vi "DataTrcFileRichInfo.vi"(9 "Language":u32, 11 "file path (dialog if empty)":path caption="文件路径 （空时为对话框）") -> (0 "路径输出":path, 1 "FileInfo":string, 2 "文件类型":string)   [LabVIEW 2015]
uses:
  <vilib>/Utility/file.llb/Read Delimited Spreadsheet (string).vi
  <vilib>/regexp/Match Regular Expression.xnode
panel:
  out "总帧数":i32
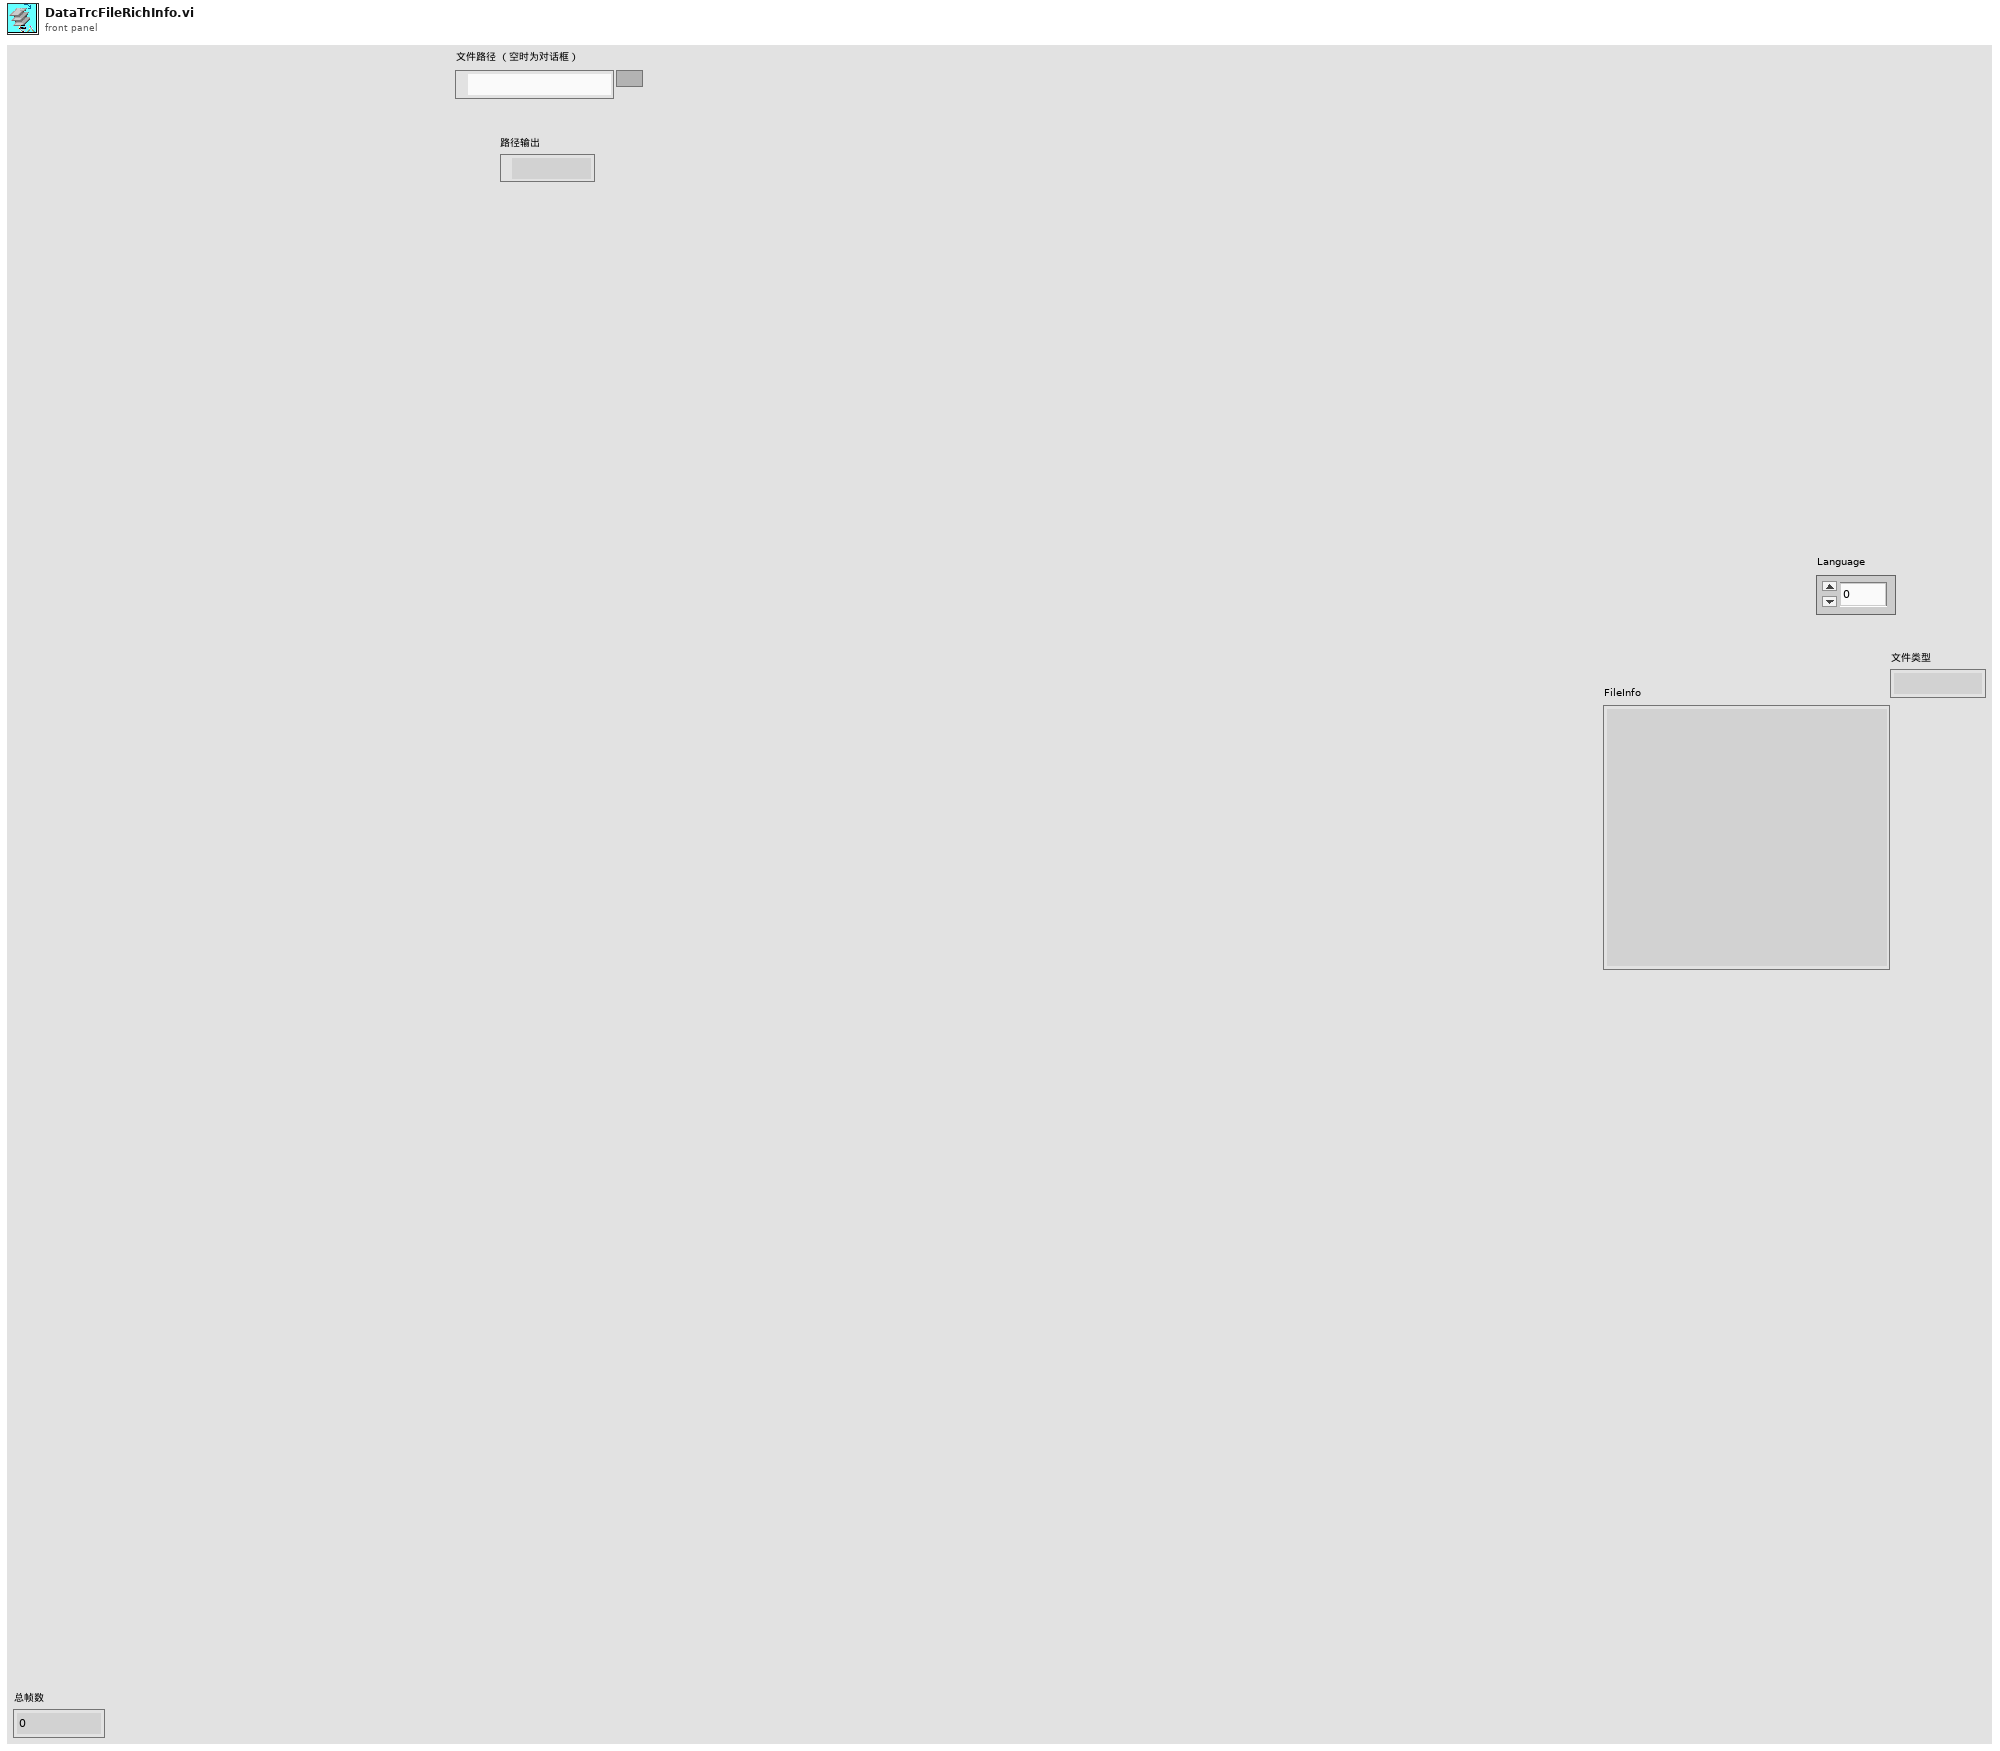
[diagram p1: front panel]
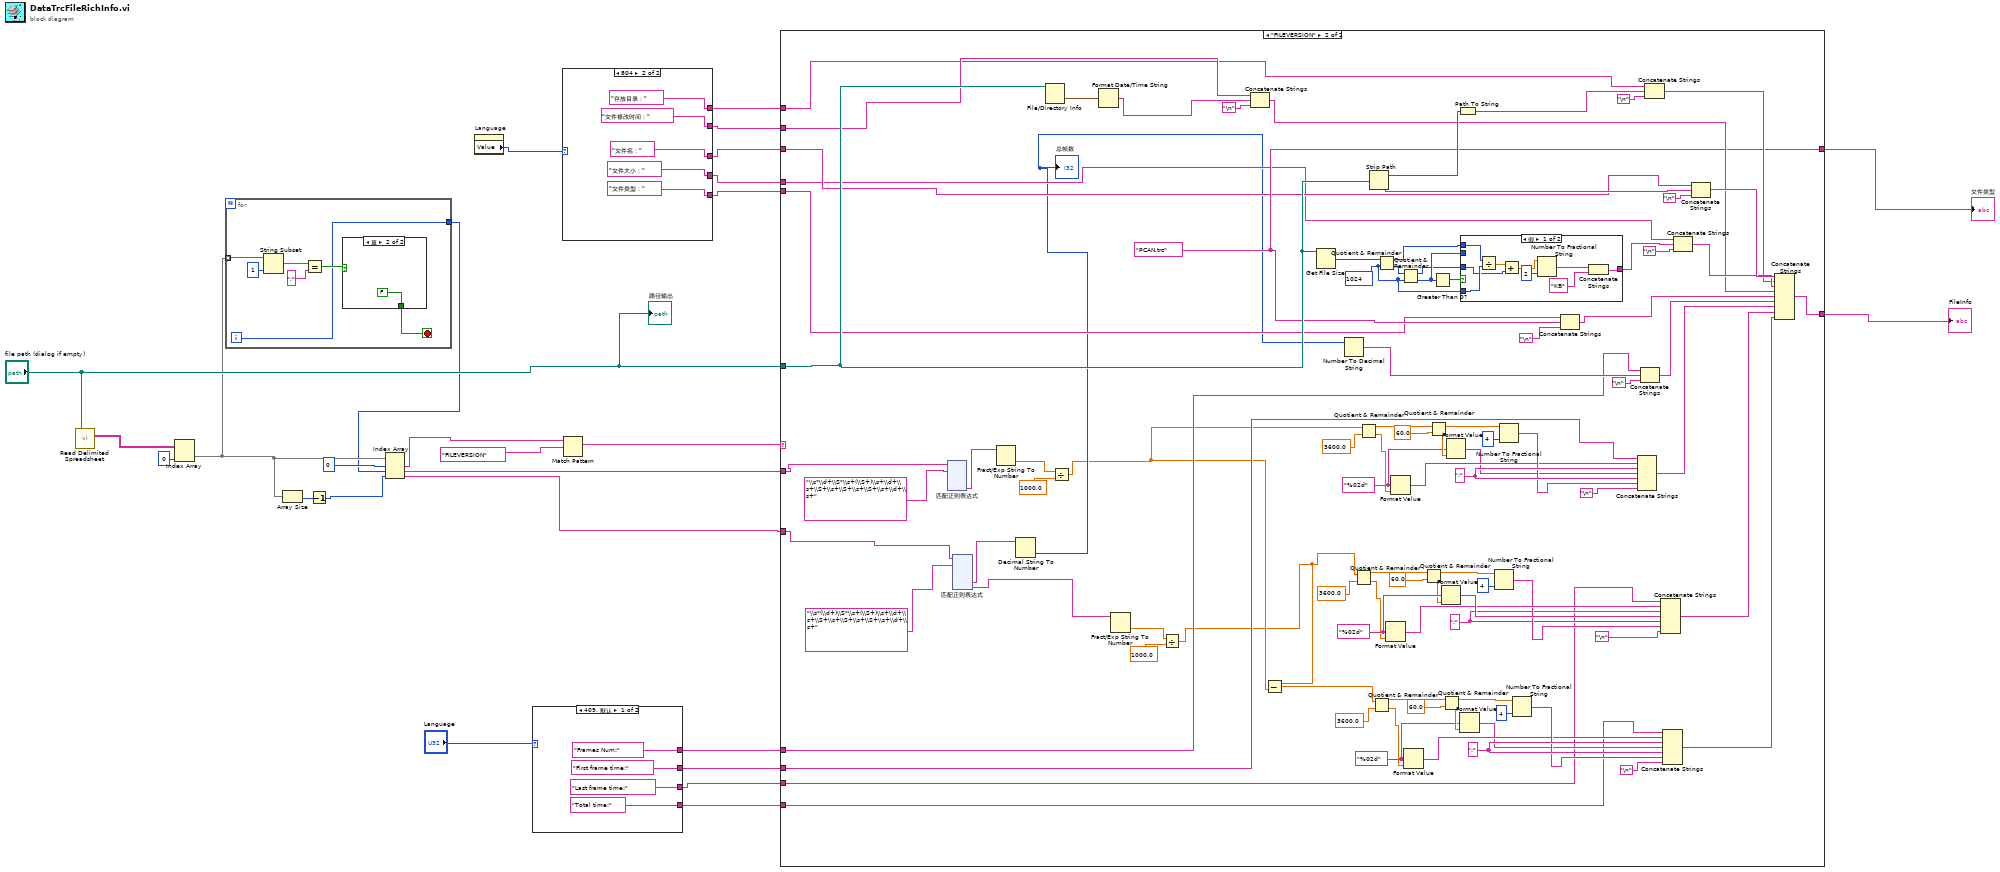
[diagram p0: block diagram]
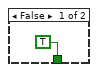
[diagram p2: hidden frame]
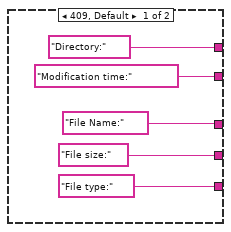
[diagram p3: hidden frame]
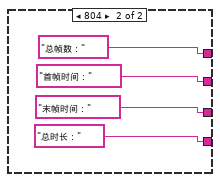
[diagram p4: hidden frame]
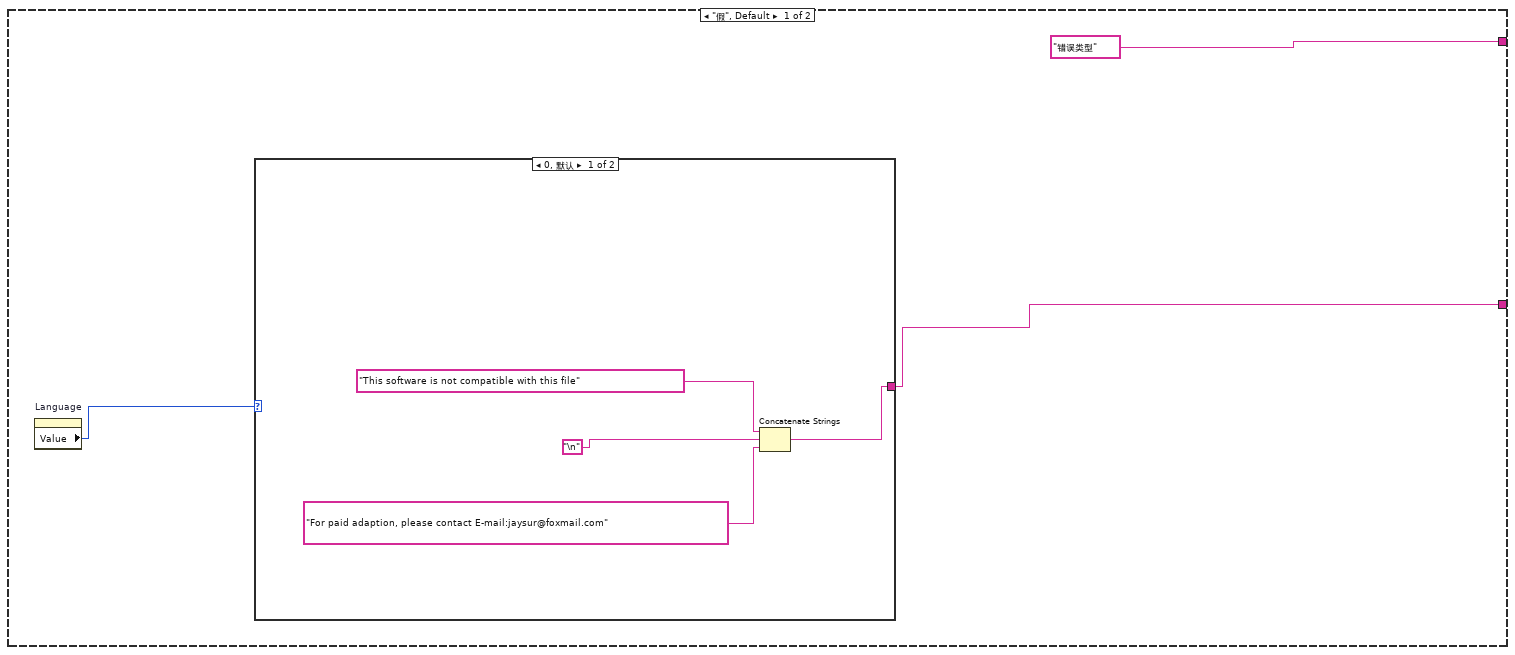
[diagram p5: hidden frame]
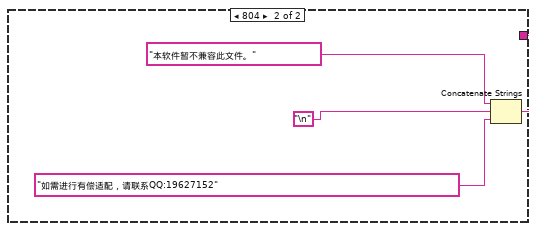
[diagram p6: hidden frame]
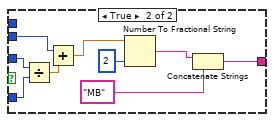
[diagram p7: hidden frame]
diagram:
  n1 = call-poly <vilib>:"Read Delimited Spreadsheet.vi"("file path (dialog if empty)"="file path (dialog if empty)") -> ("all rows"=w12:string[][])  [unwired: 9 in, 5 out]
  n2 = Index Array(array=w12, index (col)=0 ("禁用的索引 (列)")) -> (element=w3:string[])  [unwired: 1 in]
  n3 = for {
    tunnel: w3 -> [w33] mode=indexing
    tunnel: [w27] -> w2
    i -> [w27]
    stop <- w28 stop-if-true
    n4 = String Subset(string=w33, length (rest)=1 ("长度（剩余）")) -> (substring=w31:string)  [unwired: 1 in]
    n5 = Equal?(x=w31, y=";") -> (x = y?=w29:bool)
    n6 = case shown="真" w29 {
      tunnel: [TRUE FALSE] -> w28
      frame False {
      }
      frame True {
      }
    }
  }
  n7 = Array Size(array=w3) -> (size(s)=w11:i32)
  n8 = Decrement(x=w11) -> (x-1=w9:i32)
  n9 = Index Array(array=w3, index #1=0, index #2=w2, index #3=w9) -> (element #1=w7:string, element #2=w5:string, element #3=w4:string)
  n10 = property on="Language" class="DigNum (严格)"() -> ("Value"=w23:u32)  [unwired: 2 in, 2 out]
  n11 = case shown="409, 默认" "Language" {
    tunnel: ["Total time:" "总时长："] -> w17
    tunnel: ["Last frame time:" "末帧时间："] -> w16
    tunnel: ["First frame time:" "首帧时间："] -> w15
    tunnel: ["Frames Num:" "总帧数："] -> w14
    frame 409, Default {
    }
    frame 804 {
    }
  }
  n12 = case shown="804" w23 {
    tunnel: ["Modification time:" "文件修改时间："] -> w22
    tunnel: ["Directory:" "存放目录："] -> w19
    tunnel: ["File Name:" "文件名："] -> w20
    tunnel: ["File size:" "文件大小："] -> w18
    tunnel: ["File type:" "文件类型："] -> w21
    frame 409, Default {
    }
    frame 804 {
    }
  }
  n13 = Match Pattern(string=w7, regular expression="FILEVERSION" ("正则表达式")) -> (match substring=w6:string)  [unwired: 1 in, 3 out]
  n14 = case shown="\"FILEVERSION\"" w6 {
    tunnel: ["错误类型" w87] -> w26
    tunnel: [w55 w147] -> w25
    tunnel: "file path (dialog if empty)" -> [_ w90]
    tunnel: w22 -> [_ w88]
    tunnel: w21 -> [_ w86]
    tunnel: w20 -> [_ w85]
    tunnel: w19 -> [_ w84]
    tunnel: w18 -> [_ w83]
    tunnel: w17 -> [_ w82]
    tunnel: w16 -> [_ w81]
    tunnel: w15 -> [_ w80]
    tunnel: w14 -> [_ w79]
    tunnel: w5 -> [_ w77]
    tunnel: w4 -> [_ w78]
    frame "假", Default {
      n15 = property on="Language" class="DigNum (严格)"() -> ("Value"=w54:u32)  [unwired: 2 in, 2 out]
      n16 = case shown="0, 默认" w54 {
        tunnel: [w57 w61] -> w55
        frame 0, Default {
          n17 = Concatenate Strings("This software is not compatible with this file", "\n", "For paid adaption, please contact E-mail:jaysur@foxmail.com") -> (w57:string)
        }
        frame 804 {
          n18 = Concatenate Strings("本软件暂不兼容此文件。", "\n", "如需进行有偿适配，请联系QQ:19627152") -> (w61:string)
        }
      }
    }
    frame "FILEVERSION" {
      w87 = "PCAN.trc"
      w102 = i64 1024 ("y")
      w121 = "%02d" ("格式字符串")
      w127 = ":"
      w145 = "%02d" ("格式字符串")
      w139 = ":"
      w148 = "%02d" ("格式字符串")
      w154 = ":"
      n19 = xnode "匹配正则表达式"("输入字符串"=w77, "正则表达式"="\\s*\\d+\\S*\\s+(\\S+)\\s+\\d+\\s+\\S+\\s+\\S+\\s+\\S+\\s+\\d+\\s+" ("格式字符串")) -> ("子匹配 1"=w76:string)  [unwired: 4 in, 5 out]
      n20 = xnode "匹配正则表达式"("输入字符串"=w78, "正则表达式"="\\s*(\\d+)\\S*\\s+(\\S+)\\s+\\d+\\s+\\S+\\s+\\S+\\s+\\S+\\s+\\d+\\s+" ("格式字符串")) -> ("子匹配 1"=w67:string, "子匹配 2"=w68:string)  [unwired: 4 in, 5 out]
      n21 = Fract/Exp String To Number(string=w76) -> (number=w74:dbl)  [unwired: 3 in, 1 out]
      n22 = Decimal String To Number(string=w67) -> (number=w75:i32)  [unwired: 2 in, 1 out]
      "总帧数" <- w75
      n23 = File/Directory Info(path=w90) -> (last mod=w93:timestamp)  [unwired: 1 in, 6 out]
      n24 = Divide(x=w74, y=1000.0) -> (x/y=w73:dbl)
      n25 = Format Date/Time String(seconds (now)=w93) -> (date/time string=w91:string)  [unwired: 2 in]
      n26 = Fract/Exp String To Number(string=w68) -> (number=w70:dbl)  [unwired: 3 in, 1 out]
      n27 = Divide(x=w70, y=1000.0) -> (x/y=w69:dbl)
      n28 = Concatenate Strings(w88, w91, "\n") -> (w89:string)
      n29 = Subtract(x=w69, y=w73) -> (x-y=w120:dbl)
      n30 = Get File Size(file=w90) -> (size (in bytes)=w105:i64)  [unwired: 1 in, 2 out]
      n31 = Number To Decimal String(number=w75) -> (decimal integer string=w108:string)  [unwired: 1 in]
      n32 = Quotient & Remainder(x=w69, y=3600.0) -> (x-y*floor(x/y)=w135:dbl, floor(x/y)=w142:dbl)
      n33 = Quotient & Remainder(x=w73, y=3600.0) -> (x-y*floor(x/y)=w158:dbl, floor(x/y)=w151:dbl)
      n34 = Strip Path(path=w90) -> (stripped path=w95:path, name=w115:string)
      n35 = Quotient & Remainder(x=w120, y=3600.0) -> (x-y*floor(x/y)=w131:dbl, floor(x/y)=w124:dbl)
      n36 = Quotient & Remainder(x=w105, y=w102) -> (x-y*floor(x/y)=w98:i64, floor(x/y)=w104:i64)
      n37 = Format Value(format string=w145, value (0)=w142) -> (output string=w141:string)  [unwired: 1 in]
      n38 = Format Value(format string=w148, value (0)=w151) -> (output string=w152:string)  [unwired: 1 in]
      n39 = Quotient & Remainder(x=w104, y=w102) -> (x-y*floor(x/y)=w100:i64, floor(x/y)=w101:i64)
      n40 = Format Value(format string=w121, value (0)=w124) -> (output string=w125:string)  [unwired: 1 in]
      n41 = Quotient & Remainder(x=w135, y=60.0) -> (x-y*floor(x/y)=w137:dbl, floor(x/y)=w143:dbl)
      n42 = Quotient & Remainder(x=w158, y=60.0) -> (x-y*floor(x/y)=w156:dbl, floor(x/y)=w150:dbl)
      n43 = Greater Than 0?(x=w101) -> (x > 0?=w103:bool)
      n44 = Format Value(format string=w145, value (0)=w143) -> (output string=w144:string)  [unwired: 1 in]
      n45 = Quotient & Remainder(x=w131, y=60.0) -> (x-y*floor(x/y)=w129:dbl, floor(x/y)=w123:dbl)
      n46 = Format Value(format string=w148, value (0)=w150) -> (output string=w149:string)  [unwired: 1 in]
      n47 = Path To String(path=w95) -> (string=w96:string)
      n48 = Format Value(format string=w121, value (0)=w123) -> (output string=w122:string)  [unwired: 1 in]
      n49 = case shown="假" w103 {
        tunnel: w102 -> [w398 w408]
        tunnel: w101 -> [_ w406]
        tunnel: w100 -> [w396 w409]
        tunnel: [w401 w404] -> w99
        tunnel: w98 -> [w399 _]
        frame False {
          n50 = Divide(x=w399, y=w398) -> (x/y=w397:dbl)
          n51 = Add(x=w397, y=w396) -> (x+y=w395:dbl)
          n52 = Number To Fractional String(number=w395, precision (6)=i16 2 ("精度(6)")) -> (F-format string=w393:string)  [unwired: 2 in]
          n53 = Concatenate Strings(w393, "KB" ("字符串")) -> (w401:string)
        }
        frame True {
          n54 = Divide(x=w409, y=w408) -> (x/y=w407:dbl)
          n55 = Add(x=w406, y=w407) -> (x+y=w405:dbl)
          n56 = Number To Fractional String(number=w405, precision (6)=i16 2 ("精度(6)")) -> (F-format string=w403:string)  [unwired: 2 in]
          n57 = Concatenate Strings(w403, "MB") -> (w404:string)
        }
      }
      n58 = Number To Fractional String(number=w137, precision (6)=i16 4 ("精度(6)")) -> (F-format string=w140:string)  [unwired: 2 in]
      n59 = Number To Fractional String(number=w156, precision (6)=i16 4 ("精度(6)")) -> (F-format string=w153:string)  [unwired: 2 in]
      n60 = Number To Fractional String(number=w129, precision (6)=i16 4 ("精度(6)")) -> (F-format string=w126:string)  [unwired: 2 in]
      n61 = Concatenate Strings(w86, w87, "\n") -> (w112:string)
      n62 = Concatenate Strings(w80, w152, w154, w149, w154, w153, "\n") -> (w146:string)
      n63 = Concatenate Strings(w79, w108, "\n") -> (w109:string)
      n64 = Concatenate Strings(w84, w96, "\n") -> (w94:string)
      n65 = Concatenate Strings(w81, w141, w139, w144, w139, w140, "\n") -> (w133:string)
      n66 = Concatenate Strings(w82, w125, w127, w122, w127, w126, "\n") -> (w119:string)
      n67 = Concatenate Strings(w83, w99, "\n") -> (w106:string)
      n68 = Concatenate Strings(w85, w115, "\n") -> (w114:string)
      n69 = Concatenate Strings(w114, w94, w106, w89, w112, w109, w146, w133, w119) -> (w147:string)
    }
  }
  "FileInfo" <- w25
  "文件类型" <- w26
  "路径输出" <- "file path (dialog if empty)"
